vi "GlobalVariable.vi"() -> ()   [LabVIEW 2017]
panel:
  in  "format":string
  in  "csv-data":string
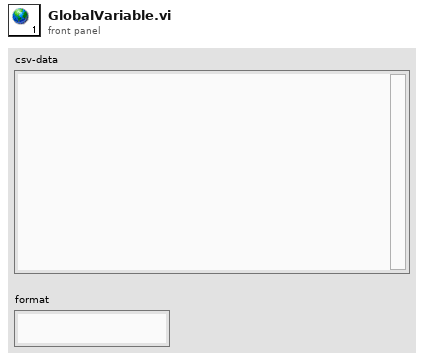
[diagram p1: front panel]
diagram:
